vi "Read Zeiss Parameters.vi"(5 "Close session":bool, 7 "Initialization":bool=TRUE, 8 "error in (no error)":errorcluster, 9 "FIB":bool=TRUE, 11 "COM port in":refnum<visa-resource-name>="COM1") -> (0 "error out":errorcluster, 1 "FIB parameters":T1, 2 "SEM parameters":T2={"Detector A"="", "Detector B"="Detecter B name", "Brightness A"=0.0, "Contrast A"=0.0, "Brightness B"=0.0, "Contrast B"=0.0, "Magnification"=0.0, "Pixel size"=0.0, "Working distance"=0.0, "EHT"=0.0, "Aperture"=0, "High current mode"=0, "Probe current"=0.0, "Scan rotation"=0.0, "Chamber vac"=0.0, "Gun vac"=0.0, "Beam shift X"=0.0, "Beam shift Y"=0.0, "Stig X"=0.0, "Stig Y"=0.0, "Alignment X"=0.0, "Alignment Y"=0.0, "Stage X"=0.0, "Stage Y"=0.0, "Stage Z"=0.0, "Stage T"=0.0, "Stage R"=0.0, "Stage M"=0.0}, 3 "COM port out":refnum<visa-resource-name>)   [LabVIEW 2018]
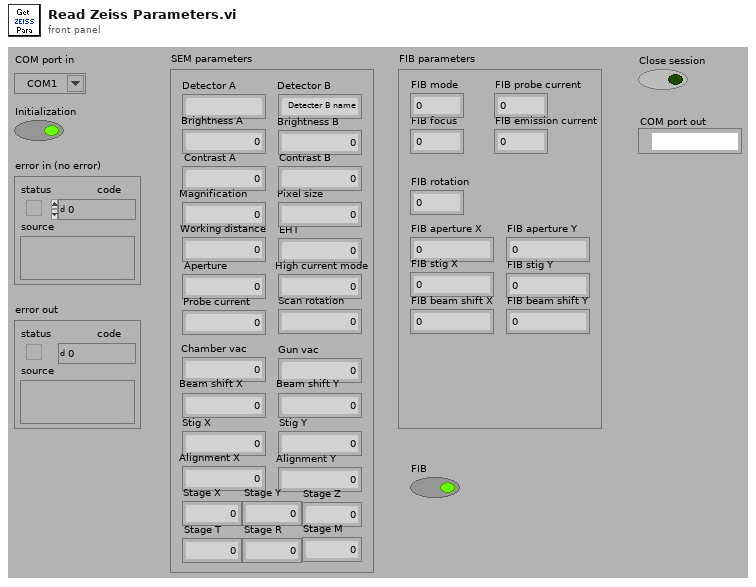
[diagram p1: front panel]
types:
  T1 = cluster{"FIB mode":u8, "FIB focus":sgl, "FIB probe current":u8, "FIB emission current":sgl, "FIB rotation":sgl, "FIB aperture X":sgl, "FIB aperture Y":sgl, "FIB stig X":sgl, "FIB stig Y":sgl, "FIB beam shift X":sgl, "FIB beam shift Y":sgl}
  T2 = cluster{"Detector A":string, "Detector B":string, "Brightness A":sgl, "Contrast A":sgl, "Brightness B":sgl, "Contrast B":sgl, "Magnification":sgl, "Pixel size":sgl, "Working distance":sgl, "EHT":sgl, "Aperture":u8, "High current mode":u8, "Probe current":sgl, "Scan rotation":sgl, "Chamber vac":sgl, "Gun vac":sgl, "Beam shift X":sgl, "Beam shift Y":sgl, "Stig X":sgl, "Stig Y":sgl, "Alignment X":sgl, "Alignment Y":sgl, "Stage X":sgl, "Stage Y":sgl, "Stage Z":sgl, "Stage T":sgl, "Stage R":sgl, "Stage M":sgl}
  T3 = cluster{"token string":string, string, sgl, sgl, "number":sgl, "number":sgl, sgl, sgl, sgl, sgl, u8, u8, sgl, sgl, sgl, sgl, sgl, sgl, sgl, sgl, sgl, sgl, sgl, sgl, sgl, sgl, sgl, sgl}
  T4 = cluster{u8, sgl, u8, sgl, sgl, sgl, sgl, sgl, sgl, sgl, sgl}
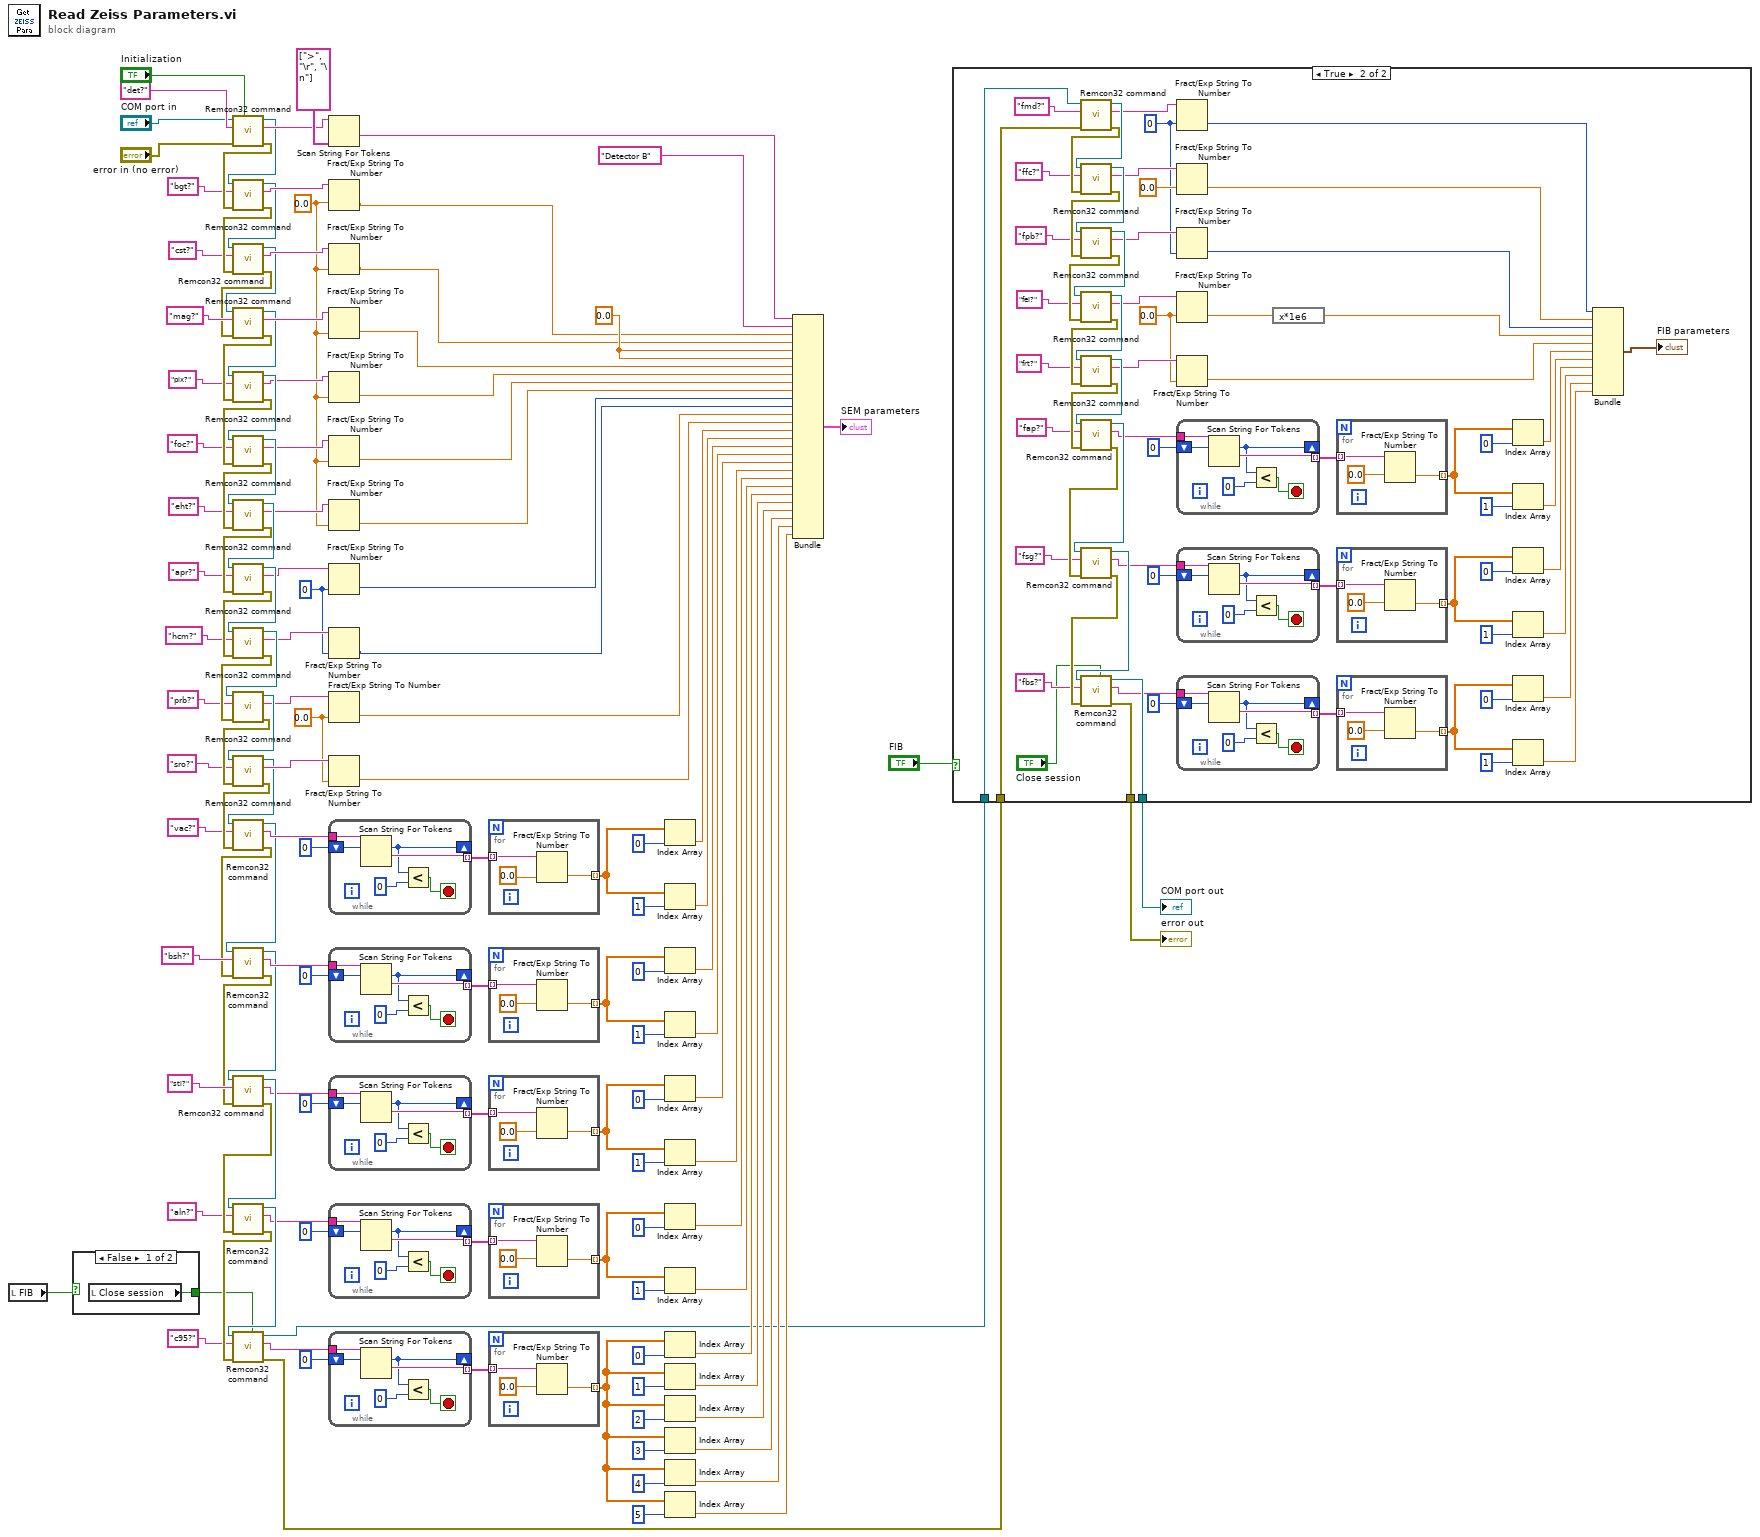
[diagram p0: block diagram]
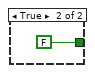
[diagram p2: hidden frame]
diagram:
  w5 = sgl 0.0 ("default (0 DBL)")
  w8 = u8 0 ("default (0 DBL)")
  (unwired) sgl 0.0 ("default (0 DBL)")
  w9 = sgl 0.0 ("default (0 DBL)")
  w92 = sgl 0.0 ("number")
  n1 = local read "FIB"() -> (w2:bool)
  n2 = case shown="False" w2 {
    tunnel: [w134 FALSE ("Close session")] -> w1
    frame False {
      n3 = local read "Close session"() -> (w134:bool)
    }
    frame True {
    }
  }
  n4 = call "Remcon32 command.vi"("Initialization"="Initialization", "error in"="error in (no error)", "SEM command"="det?" ("write buffer"), "COM port in"="COM port in") -> ("error out"=w85:errorcluster, "SEM reply"=w87:string, "COM port out"=w86:refnum<visa-resource-name>)  [unwired: 1 in, 4 out]
  n5 = call "Remcon32 command.vi"("error in"=w85, "SEM command"="bgt?" ("write buffer"), "COM port in"=w86) -> ("error out"=w81:errorcluster, "SEM reply"=w83:string, "COM port out"=w82:refnum<visa-resource-name>)  [unwired: 2 in, 4 out]
  n6 = call "Remcon32 command.vi"("error in"=w81, "SEM command"="cst?" ("write buffer"), "COM port in"=w82) -> ("error out"=w76:errorcluster, "SEM reply"=w79:string, "COM port out"=w77:refnum<visa-resource-name>)  [unwired: 2 in, 4 out]
  n7 = call "Remcon32 command.vi"("error in"=w76, "SEM command"="mag?" ("write buffer"), "COM port in"=w77) -> ("error out"=w74:errorcluster, "SEM reply"=w75:string, "COM port out"=w73:refnum<visa-resource-name>)  [unwired: 2 in, 4 out]
  n8 = call "Remcon32 command.vi"("error in"=w74, "SEM command"="pix?" ("write buffer"), "COM port in"=w73) -> ("error out"=w71:errorcluster, "SEM reply"=w53:string, "COM port out"=w72:refnum<visa-resource-name>)  [unwired: 2 in, 4 out]
  n9 = call "Remcon32 command.vi"("error in"=w71, "SEM command"="foc?" ("write buffer"), "COM port in"=w72) -> ("error out"=w69:errorcluster, "SEM reply"=w50:string, "COM port out"=w70:refnum<visa-resource-name>)  [unwired: 2 in, 4 out]
  n10 = call "Remcon32 command.vi"("error in"=w69, "SEM command"="eht?" ("write buffer"), "COM port in"=w70) -> ("error out"=w67:errorcluster, "SEM reply"=w51:string, "COM port out"=w68:refnum<visa-resource-name>)  [unwired: 2 in, 4 out]
  n11 = call "Remcon32 command.vi"("error in"=w67, "SEM command"="apr?" ("write buffer"), "COM port in"=w68) -> ("error out"=w65:errorcluster, "SEM reply"=w52:string, "COM port out"=w66:refnum<visa-resource-name>)  [unwired: 2 in, 4 out]
  n12 = call "Remcon32 command.vi"("error in"=w65, "SEM command"="hcm?" ("write buffer"), "COM port in"=w66) -> ("error out"=w63:errorcluster, "SEM reply"=w49:string, "COM port out"=w64:refnum<visa-resource-name>)  [unwired: 2 in, 4 out]
  n13 = call "Remcon32 command.vi"("error in"=w63, "SEM command"="prb?" ("write buffer"), "COM port in"=w64) -> ("error out"=w61:errorcluster, "SEM reply"=w48:string, "COM port out"=w62:refnum<visa-resource-name>)  [unwired: 2 in, 4 out]
  n14 = call "Remcon32 command.vi"("error in"=w61, "SEM command"="sro?" ("write buffer"), "COM port in"=w62) -> ("error out"=w42:errorcluster, "SEM reply"=w47:string, "COM port out"=w41:refnum<visa-resource-name>)  [unwired: 2 in, 4 out]
  n15 = call "Remcon32 command.vi"("error in"=w42, "SEM command"="vac?" ("write buffer"), "COM port in"=w41) -> ("error out"=w15:errorcluster, "SEM reply"=w36:string, "COM port out"=w17:refnum<visa-resource-name>)  [unwired: 2 in, 4 out]
  n16 = call "Remcon32 command.vi"("error in"=w15, "SEM command"="bsh?" ("write buffer"), "COM port in"=w17) -> ("error out"=w14:errorcluster, "SEM reply"=w23:string, "COM port out"=w16:refnum<visa-resource-name>)  [unwired: 2 in, 4 out]
  n17 = call "Remcon32 command.vi"("error in"=w14, "SEM command"="sti?" ("write buffer"), "COM port in"=w16) -> ("error out"=w45:errorcluster, "SEM reply"=w35:string, "COM port out"=w46:refnum<visa-resource-name>)  [unwired: 2 in, 4 out]
  n18 = call "Remcon32 command.vi"("error in"=w45, "SEM command"="aln?" ("write buffer"), "COM port in"=w46) -> ("error out"=w43:errorcluster, "SEM reply"=w34:string, "COM port out"=w44:refnum<visa-resource-name>)  [unwired: 2 in, 4 out]
  n19 = call "Remcon32 command.vi"("Close session"=w1, "error in"=w43, "SEM command"="c95?" ("write buffer"), "COM port in"=w44) -> ("error out"=w31:errorcluster, "SEM reply"=w33:string, "COM port out"=w32:refnum<visa-resource-name>)  [unwired: 1 in, 4 out]
  n20 = Scan String For Tokens(6:string[] [">", "\r", "\n"] ("delimiters (\\s,\\t,\\r,\\n)"), 9:w87) -> (1:w94:string)  [unwired: 1 in, 6 out]
  n21 = Fract/Exp String To Number(string=w83, default (0 dbl)=w9) -> (number=w10:sgl)  [unwired: 3 out]
  n22 = Fract/Exp String To Number(string=w79, default (0 dbl)=w9) -> (number=w11:sgl)  [unwired: 3 out]
  n23 = Fract/Exp String To Number(string=w75, default (0 dbl)=w9) -> (number=w96:sgl)  [unwired: 3 out]
  n24 = Fract/Exp String To Number(string=w53, default (0 dbl)=w9) -> (number=w97:sgl)  [unwired: 3 out]
  n25 = Fract/Exp String To Number(string=w50, default (0 dbl)=w9) -> (number=w98:sgl)  [unwired: 3 out]
  n26 = Fract/Exp String To Number(string=w51, default (0 dbl)=w9) -> (number=w99:sgl)  [unwired: 3 out]
  n27 = Fract/Exp String To Number(string=w52, default (0 dbl)=w8) -> (number=w7:u8)  [unwired: 3 out]
  n28 = Fract/Exp String To Number(string=w49, default (0 dbl)=w8) -> (number=w6:u8)  [unwired: 3 out]
  n29 = Fract/Exp String To Number(string=w48, default (0 dbl)=w5) -> (number=w100:sgl)  [unwired: 3 out]
  n30 = Fract/Exp String To Number(string=w47, default (0 dbl)=w5) -> (number=w101:sgl)  [unwired: 3 out]
  n31 = while {
    shift-right: [w138] -> _
    shift-left: 0 ("offset past token") -> [w141]
    tunnel: [w139] -> w125 mode=indexing
    tunnel: w36 -> [w136]
    stop <- w137 stop-if-true
    n32 = Scan String For Tokens(8:w141, 9:w136) -> (1:w139:string, 2:w138:i32)  [unwired: 1 in, 5 out]
    n33 = Less?(x=w138, y=0) -> (x < y?=w137:bool)
  }
  n34 = while {
    shift-right: [w144] -> _
    shift-left: 0 ("offset past token") -> [w147]
    tunnel: [w145] -> w18 mode=indexing
    tunnel: w23 -> [w142]
    stop <- w143 stop-if-true
    n35 = Scan String For Tokens(8:w147, 9:w142) -> (1:w145:string, 2:w144:i32)  [unwired: 1 in, 5 out]
    n36 = Less?(x=w144, y=0) -> (x < y?=w143:bool)
  }
  n37 = while {
    shift-right: [w150] -> _
    shift-left: 0 ("offset past token") -> [w153]
    tunnel: [w151] -> w133 mode=indexing
    tunnel: w35 -> [w148]
    stop <- w149 stop-if-true
    n38 = Scan String For Tokens(8:w153, 9:w148) -> (1:w151:string, 2:w150:i32)  [unwired: 1 in, 5 out]
    n39 = Less?(x=w150, y=0) -> (x < y?=w149:bool)
  }
  n40 = while {
    shift-right: [w156] -> _
    shift-left: 0 ("offset past token") -> [w159]
    tunnel: [w157] -> w129 mode=indexing
    tunnel: w34 -> [w154]
    stop <- w155 stop-if-true
    n41 = Scan String For Tokens(8:w159, 9:w154) -> (1:w157:string, 2:w156:i32)  [unwired: 1 in, 5 out]
    n42 = Less?(x=w156, y=0) -> (x < y?=w155:bool)
  }
  n43 = while {
    shift-right: [w162] -> _
    shift-left: 0 ("offset past token") -> [w165]
    tunnel: [w163] -> w115 mode=indexing
    tunnel: w33 -> [w160]
    stop <- w161 stop-if-true
    n44 = Scan String For Tokens(8:w165, 9:w160) -> (1:w163:string, 2:w162:i32)  [unwired: 1 in, 5 out]
    n45 = Less?(x=w162, y=0) -> (x < y?=w161:bool)
  }
  n46 = for {
    tunnel: w125 -> [w168] mode=indexing
    tunnel: [w167] -> w124 mode=indexing
    n47 = Fract/Exp String To Number(string=w168, default (0 dbl)=sgl 0.0 ("default (0 DBL)")) -> (number=w167:sgl)  [unwired: 3 out]
  }
  n48 = for {
    tunnel: w18 -> [w171] mode=indexing
    tunnel: [w170] -> w19 mode=indexing
    n49 = Fract/Exp String To Number(string=w171, default (0 dbl)=sgl 0.0 ("default (0 DBL)")) -> (number=w170:sgl)  [unwired: 3 out]
  }
  n50 = for {
    tunnel: w133 -> [w174] mode=indexing
    tunnel: [w173] -> w132 mode=indexing
    n51 = Fract/Exp String To Number(string=w174, default (0 dbl)=sgl 0.0 ("default (0 DBL)")) -> (number=w173:sgl)  [unwired: 3 out]
  }
  n52 = for {
    tunnel: w129 -> [w177] mode=indexing
    tunnel: [w176] -> w128 mode=indexing
    n53 = Fract/Exp String To Number(string=w177, default (0 dbl)=sgl 0.0 ("default (0 DBL)")) -> (number=w176:sgl)  [unwired: 3 out]
  }
  n54 = for {
    tunnel: w115 -> [w180] mode=indexing
    tunnel: [w179] -> w108 mode=indexing
    n55 = Fract/Exp String To Number(string=w180, default (0 dbl)=sgl 0.0 ("default (0 DBL)")) -> (number=w179:sgl)  [unwired: 3 out]
  }
  n56 = Index Array(array=w124, index=0) -> (element=w121:sgl)
  n57 = Index Array(array=w124, index=1) -> (element=w120:sgl)
  n58 = Index Array(array=w19, index=0) -> (element=w13:sgl)
  n59 = Index Array(array=w19, index=1) -> (element=w12:sgl)
  n60 = Index Array(array=w132, index=0) -> (element=w119:sgl)
  n61 = Index Array(array=w132, index=1) -> (element=w118:sgl)
  n62 = Index Array(array=w128, index=0) -> (element=w117:sgl)
  n63 = Index Array(array=w128, index=1) -> (element=w116:sgl)
  n64 = Index Array(array=w108, index=0) -> (element=w107:sgl)
  n65 = Index Array(array=w108, index=1) -> (element=w106:sgl)
  n66 = Index Array(array=w108, index=2) -> (element=w105:sgl)
  n67 = Index Array(array=w108, index=3) -> (element=w104:sgl)
  n68 = Index Array(array=w108, index=4) -> (element=w103:sgl)
  n69 = Index Array(array=w108, index=5) -> (element=w102:sgl)
  n70 = Bundle("token string"=w94, "Detector B", w10, w11, "number"=w92, "number"=w92, w96, w97, w98, w99, w7, w6, w100, w101, w121, w120, w13, w12, w119, w118, w117, w116, w107, w106, w105, w104, w103, w102) -> (→"SEM parameters":T3)  [unwired: 1 out]
  n71 = case shown="True" "FIB" {
    tunnel: w32 -> [w181 w202]
    tunnel: w31 -> [w182 w201]
    tunnel: [w181 w200] -> w30
    tunnel: [w182 w199] -> w29
    frame False {
    }
    frame True {
      w187 = sgl 0.0 ("number")
      w185 = u8 0 ("number")
      n72 = call "Remcon32 command.vi"("error in"=w201, "SEM command"="fmd?" ("write buffer"), "COM port in"=w202) -> ("error out"=w224:errorcluster, "SEM reply"=w191:string, "COM port out"=w225:refnum<visa-resource-name>)  [unwired: 2 in, 4 out]
      n73 = call "Remcon32 command.vi"("error in"=w224, "SEM command"="ffc?" ("write buffer"), "COM port in"=w225) -> ("error out"=w222:errorcluster, "SEM reply"=w192:string, "COM port out"=w223:refnum<visa-resource-name>)  [unwired: 2 in, 4 out]
      n74 = call "Remcon32 command.vi"("error in"=w222, "SEM command"="fpb?" ("write buffer"), "COM port in"=w223) -> ("error out"=w220:errorcluster, "SEM reply"=w193:string, "COM port out"=w221:refnum<visa-resource-name>)  [unwired: 2 in, 4 out]
      n75 = call "Remcon32 command.vi"("error in"=w220, "SEM command"="fei?" ("write buffer"), "COM port in"=w221) -> ("error out"=w218:errorcluster, "SEM reply"=w194:string, "COM port out"=w219:refnum<visa-resource-name>)  [unwired: 2 in, 4 out]
      n76 = call "Remcon32 command.vi"("error in"=w218, "SEM command"="frt?" ("write buffer"), "COM port in"=w219) -> ("error out"=w213:errorcluster, "SEM reply"=w195:string, "COM port out"=w212:refnum<visa-resource-name>)  [unwired: 2 in, 4 out]
      n77 = call "Remcon32 command.vi"("error in"=w213, "SEM command"="fap?" ("write buffer"), "COM port in"=w212) -> ("error out"=w216:errorcluster, "SEM reply"=w196:string, "COM port out"=w217:refnum<visa-resource-name>)  [unwired: 2 in, 4 out]
      n78 = call "Remcon32 command.vi"("error in"=w216, "SEM command"="fsg?" ("write buffer"), "COM port in"=w217) -> ("error out"=w214:errorcluster, "SEM reply"=w198:string, "COM port out"=w215:refnum<visa-resource-name>)  [unwired: 2 in, 4 out]
      n79 = call "Remcon32 command.vi"("Close session"="Close session", "error in"=w214, "SEM command"="fbs?" ("write buffer"), "COM port in"=w215) -> ("error out"=w199:errorcluster, "SEM reply"=w197:string, "COM port out"=w200:refnum<visa-resource-name>)  [unwired: 1 in, 4 out]
      n80 = Fract/Exp String To Number(string=w191, default (0 dbl)=w185) -> (number=w236:u8)  [unwired: 3 out]
      n81 = Fract/Exp String To Number(string=w192, default (0 dbl)=sgl 0.0 ("number")) -> (number=w235:sgl)  [unwired: 3 out]
      n82 = Fract/Exp String To Number(string=w193, default (0 dbl)=w185) -> (number=w234:u8)  [unwired: 3 out]
      n83 = Fract/Exp String To Number(string=w194, default (0 dbl)=w187) -> (number=w233:sgl)  [unwired: 3 out]
      n84 = Fract/Exp String To Number(string=w195, default (0 dbl)=w187) -> (number=w232:sgl)  [unwired: 3 out]
      n85 = while {
        shift-right: [w254] -> _
        shift-left: 0 ("offset past token") -> [w257]
        tunnel: [w255] -> w240 mode=indexing
        tunnel: w196 -> [w252]
        stop <- w253 stop-if-true
        n86 = Scan String For Tokens(8:w257, 9:w252) -> (1:w255:string, 2:w254:i32)  [unwired: 1 in, 5 out]
        n87 = Less?(x=w254, y=0) -> (x < y?=w253:bool)
      }
      n88 = while {
        shift-right: [w272] -> _
        shift-left: 0 ("offset past token") -> [w275]
        tunnel: [w273] -> w248 mode=indexing
        tunnel: w198 -> [w270]
        stop <- w271 stop-if-true
        n89 = Scan String For Tokens(8:w275, 9:w270) -> (1:w273:string, 2:w272:i32)  [unwired: 1 in, 5 out]
        n90 = Less?(x=w272, y=0) -> (x < y?=w271:bool)
      }
      n91 = while {
        shift-right: [w263] -> _
        shift-left: 0 ("offset past token") -> [w266]
        tunnel: [w264] -> w244 mode=indexing
        tunnel: w197 -> [w261]
        stop <- w262 stop-if-true
        n92 = Scan String For Tokens(8:w266, 9:w261) -> (1:w264:string, 2:w263:i32)  [unwired: 1 in, 5 out]
        n93 = Less?(x=w263, y=0) -> (x < y?=w262:bool)
      }
      n94 = expression code="x*1e6"(w233) -> (w183:sgl)
      n95 = for {
        tunnel: w240 -> [w251] mode=indexing
        tunnel: [w250] -> w239 mode=indexing
        n96 = Fract/Exp String To Number(string=w251, default (0 dbl)=sgl 0.0 ("number")) -> (number=w250:sgl)  [unwired: 3 out]
      }
      n97 = for {
        tunnel: w248 -> [w269] mode=indexing
        tunnel: [w268] -> w247 mode=indexing
        n98 = Fract/Exp String To Number(string=w269, default (0 dbl)=sgl 0.0 ("number")) -> (number=w268:sgl)  [unwired: 3 out]
      }
      n99 = for {
        tunnel: w244 -> [w260] mode=indexing
        tunnel: [w259] -> w243 mode=indexing
        n100 = Fract/Exp String To Number(string=w260, default (0 dbl)=sgl 0.0 ("number")) -> (number=w259:sgl)  [unwired: 3 out]
      }
      n101 = Index Array(array=w239, index=0) -> (element=w231:sgl)
      n102 = Index Array(array=w239, index=1) -> (element=w230:sgl)
      n103 = Index Array(array=w247, index=0) -> (element=w229:sgl)
      n104 = Index Array(array=w247, index=1) -> (element=w228:sgl)
      n105 = Index Array(array=w243, index=0) -> (element=w227:sgl)
      n106 = Index Array(array=w243, index=1) -> (element=w226:sgl)
      n107 = Bundle(w236, w235, w234, w183, w232, w231, w230, w229, w228, w227, w226) -> (→"FIB parameters":T4)  [unwired: 1 out]
    }
  }
  "error out" <- w29
  "COM port out" <- w30
